vi "Main.vi"() -> ()   [LabVIEW 2018]
panel:
  out "x/y":dbl
  out "숫자형 5":dbl format="%#_13g"
  in  "숫자형 4":dbl format="%#_13g"
  in  "숫자형 3":dbl format="%#_13g"
  in  "숫자형 2":dbl format="%#_13g"
  in  "숫자형":dbl format="%#_13g"
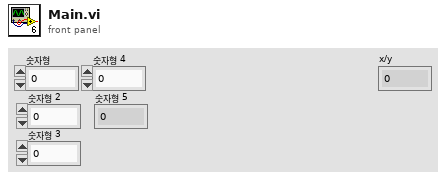
[diagram p1: front panel]
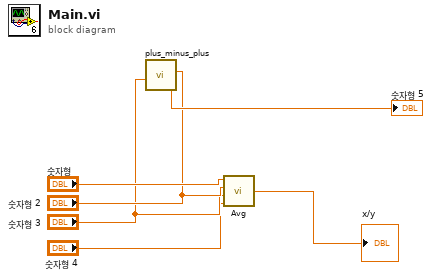
[diagram p0: block diagram]
diagram:
  n1 = call "plus_minus_plus.vi"("3"="숫자형 3", "2"="숫자형 2") -> ("숫자형 출력"=→"숫자형 5":dbl)  [unwired: 2 in]
  n2 = call "Avg.vi"("숫자형 4"="숫자형 4", "숫자형 3"="숫자형 3", "숫자형 2"="숫자형 2", "숫자형 1"="숫자형") -> ("x/y"=→"x/y":dbl)
